vi "Press2Depth.vi"(1 "Pressure in dbars":dbl) -> (0 "Depth in meters":dbl)   [LabVIEW 2014]
panel:
  out "gam_dash":dbl format="%#_10g"
  out "c1":dbl format="%#_10g"
  out "c4":dbl format="%#_10g"
  out "c3":dbl format="%#_10g"
  out "c2":dbl format="%#_10g"
  out "g":dbl format="%#_10g"
  # "Constants"
  # "This conversion is based on sw_dpth from the MATLAB seawater\npackage with latitude = 0."
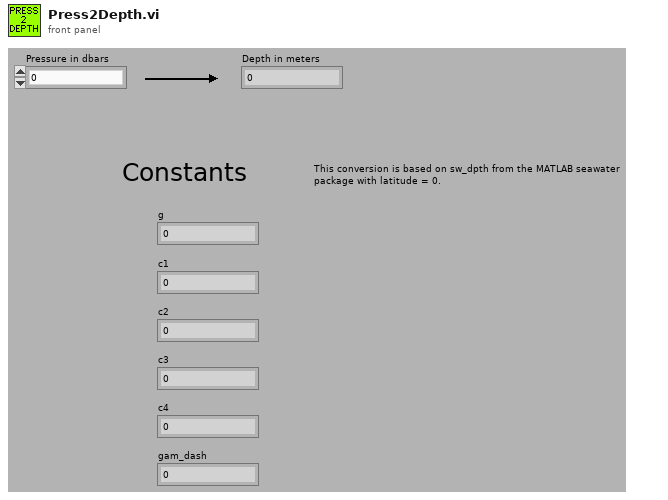
[diagram p1: front panel]
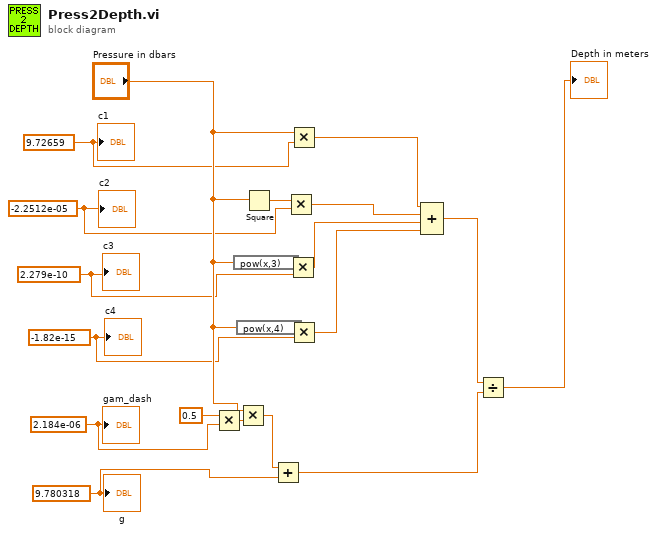
[diagram p0: block diagram]
diagram:
  w4 = 9.780318
  w5 = 2.184e-06
  w3 = -1.82e-15
  w2 = 2.279e-10
  w1 = -2.2512e-05
  w6 = 9.72659
  n1 = Multiply(x=0.5, y=w5) -> (x*y=w11:dbl)
  n2 = expression code="pow(x,3)"("Pressure in dbars") -> (w19:dbl)
  n3 = expression code="pow(x,4)"("Pressure in dbars") -> (w18:dbl)
  n4 = Multiply(x="Pressure in dbars", y=w11) -> (x*y=w9:dbl)
  n5 = Square(x="Pressure in dbars") -> (x^2=w20:dbl)
  n6 = Add(x=w9, y=w4) -> (x+y=w8:dbl)
  n7 = Multiply(x=w20, y=w1) -> (x*y=w16:dbl)
  n8 = Multiply(x=w19, y=w2) -> (x*y=w15:dbl)
  n9 = Multiply(x="Pressure in dbars", y=w6) -> (x*y=w17:dbl)
  n10 = Multiply(x=w18, y=w3) -> (x*y=w14:dbl)
  n11 = Compound Arithmetic op=ADD(w17, w16, w15, w14) -> (w13:dbl)
  n12 = Divide(x=w13, y=w8) -> (x/y=→"Depth in meters":dbl)
  "g" <- w4
  "c2" <- w1
  "c3" <- w2
  "c4" <- w3
  "c1" <- w6
  "gam_dash" <- w5
